vi "SD_Construct_data_string.vi"(4 "Line End":u16(ring)=4 items=["Nothing", "Tab", "CR", "LF", "CRLF"], 6 "Line Start":u16(ring) items=["Nothing", "Tab"], 7 "Variables to send":T1[](array[typedef])=[enum."timestamp (SW)", enum."R", enum."phi", enum."alpha", enum."X", enum."Y", enum."Zone #", enum."Speed, mm/s"], 8 "error in (no error)":errorcluster, 10 "Mode":bool, 11 "Send Frame Argument":T2 {"Data in"."Measurements and statistics"."Running, perc. of time" format="%05.2f"}) -> (0 "error out":errorcluster, 2 "Total bytes":i32, 3 "Data string":string)   [LabVIEW 2018, in "Stream Data.lvlib"]
uses:
  Stream Data.lvlib
  Send Frame Argument--cluster.ctl
  SubVi's/Controls/CTL_Full_data_frame.ctl
  SubVi's/Controls/CTL_Animal_Coordinates_and_Speed.ctl
  SubVi's/Controls/CTL_Measurements_and_Statistics.ctl
  Typedefs/CTL_Variable_to_pass.ctl
  Tracker.lvlib
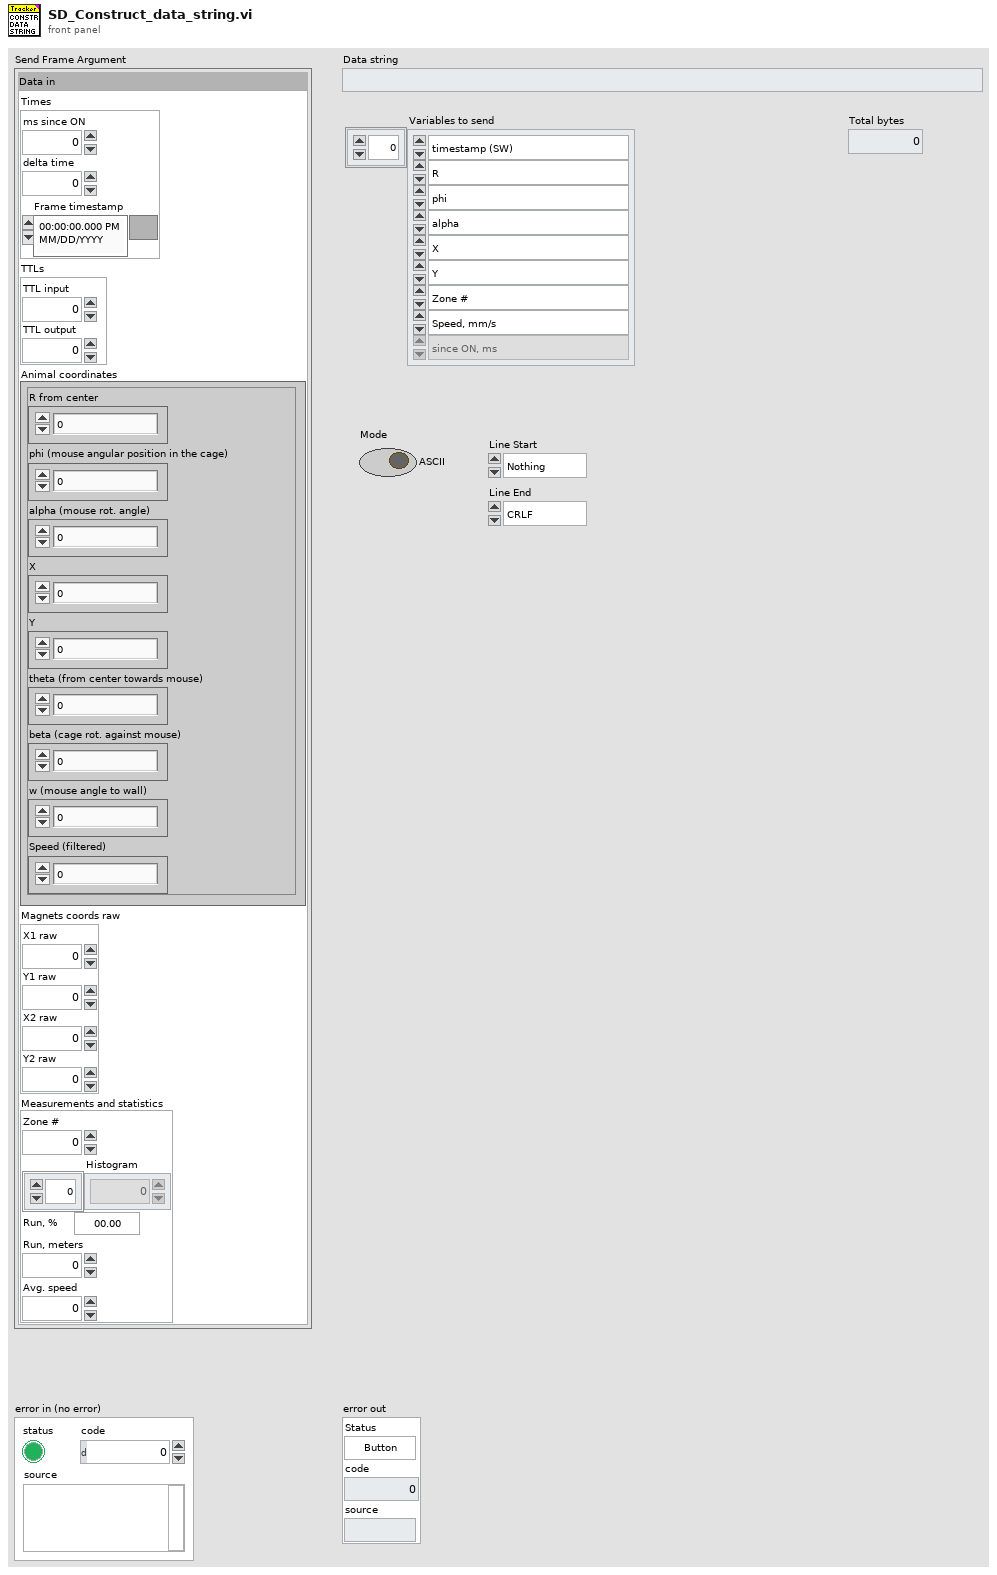
[diagram p1: front panel]
types:
  T1 = typedef "Stream Data.lvlib/CTL_Variable_to_pass.ctl" = enum16{"since ON, ms", "delta time, ms", "timestamp (SW)", "R", "phi", "alpha", "X", "Y", "Zone #", "Run percentage", "Speed, mm/s"}
  T2 = typedef "Stream Data.lvlib/Send Frame Argument--cluster.ctl" = cluster{"Data in":T3}
  T3 = typedef "Tracker.lvlib/CTL_Full_data_frame.ctl" = cluster{"Times":cluster{"ms since ON":u32, "delta time":u32, "Frame timestamp":timestamp}, "TTLs":cluster{"TTL input":i16, "TTL output":i16}, "Animal coordinates":T4, "Magnets coords raw":cluster{"X1 raw":dbl, "Y1 raw":dbl, "X2 raw":dbl, "Y2 raw":dbl}, "Measurements and statistics":T5}
  T4 = typedef "Tracker.lvlib/CTL_Animal_Coordinates_and_Speed.ctl" = cluster{"R from center":dbl, "phi (mouse angular position in the cage)":dbl, "alpha (mouse rot. angle)":dbl, "X":dbl, "Y":dbl, "theta (from center towards mouse)":dbl, "beta (cage rot. against mouse)":dbl, "w (mouse angle to wall)":dbl, "Speed (filtered)":dbl}
  T5 = typedef "Tracker.lvlib/CTL_Measurements_and_Statistics.ctl" = cluster{"Zone #":i8, "Histogram":dbl[], "Running, perc. of time":dbl, "Run, meters":dbl, "Avg. speed":dbl}
  T6 = enum16{"big-endian, network order", "native, host order", "little-endian"}
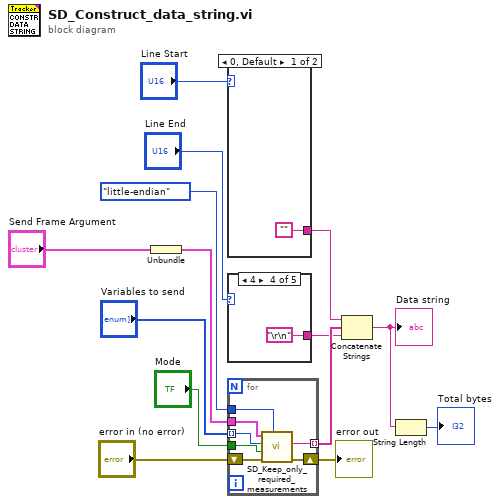
[diagram p0: block diagram]
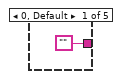
[diagram p2: hidden frame]
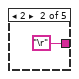
[diagram p3: hidden frame]
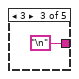
[diagram p4: hidden frame]
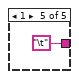
[diagram p5: hidden frame]
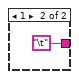
[diagram p6: hidden frame]
diagram:
  n1 = Unbundle("Send Frame Argument") -> ("Data in"=w11:T3)
  n2 = case shown="0, Default" "Line Start" {
    tunnel: ["" "\t"] -> w6
    frame 0, Default {
    }
    frame 1 {
    }
  }
  n3 = case shown="4" "Line End" {
    tunnel: ["" "\r" "\n" "\r\n" "\t"] -> w4
    frame 0, Default {
    }
    frame 2 {
    }
    frame 3 {
    }
    frame 4 {
    }
    frame 1 {
    }
  }
  n4 = for {
    tunnel: "Variables to send" -> [w28] mode=indexing
    tunnel: "Mode" -> [w27]
    tunnel: w11 -> [w26]
    tunnel: [w25] -> w7 mode=indexing
    shift-right: [w23] -> w9
    shift-left: "error in (no error)" -> [w24]
    tunnel: T6."little-endian" ("byte order") -> [w22]
    n5 = call "SD_Keep_only_required_measurements.vi"("byte order"=w22, "error in (no error)"=w24, "Mode"=w27, "Variable"=w28, "Data in"=w26) -> ("error out"=w23:errorcluster, "Data string"=w25:string)  [unwired: 3 in, 2 out]
  }
  "error out" <- w9
  n6 = Concatenate Strings(w6, w7, w4) -> (w2:string)
  "Data string" <- w2
  n7 = String Length(string=w2) -> (length=→"Total bytes":i32)
